vi "Untitled 21 (SubVI).vi"(6 "passband bandwidth (Hz)":dbl, 7 "pulse shaping filter (none) in":T1(ring), 9 "carrier frequency (Hz) in":dbl, 10 "Numeric":i32, 11 "passband waveform":waveform(dbl)) -> (3 "output bit stream":i8[](array[numeric]))   [LabVIEW 2017]
uses:
  <vilib>/addons/Modulation/Analog/support/mod_Set Error Source.vi
  <vilib>/addons/Modulation/Digital/General/MT Generate ASK system parameters (M).vi
  <vilib>/addons/Modulation/Digital/Support/Common/Validators/mod_Generate Filter Coefficients Validate.vi
  <vilib>/addons/Modulation/Digital/General/subVIs/mod_Generate Filter Coefficients.vi
  <vilib>/addons/Modulation/Analog/MT Downconvert Passband (Real).vi
  <vilib>/addons/Modulation/niDMT.lvlib
  <vilib>/addons/Modulation/niAMT.lvlib
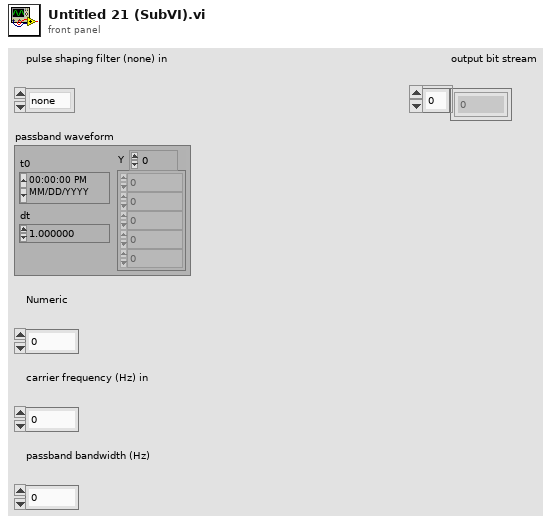
[diagram p1: front panel]
types:
  T1 = enum16{"none", "Raised Cosine", "Root Raised Cos", "Gaussian"}
  T2 = enum16{"FSK", "PSK", "QAM", "MSK", "PAM", "ASK", "CPM"}
  T3 = typedef "niAMT.lvlib/Complex Data Waveform.ctl" = cluster{"t0":dbl, "dt":dbl, "Y":cdb[]}
  T4 = cluster{"samples per symbol (16)":i32, "symbol map":cdb[]}
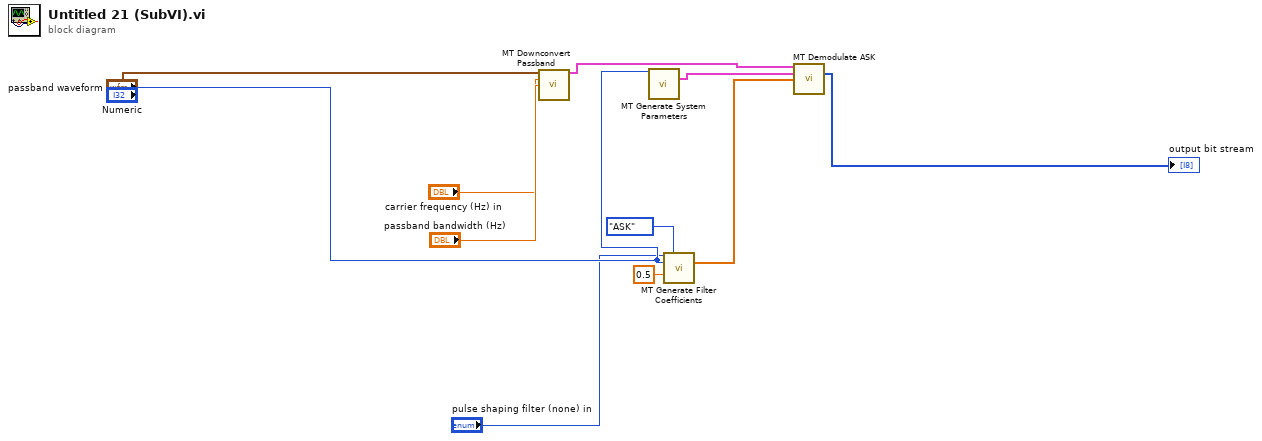
[diagram p0: block diagram]
diagram:
  n1 = call-poly <vilib>:"MT Downconvert Passband.vi"("Waveform"="passband waveform", "carrier frequency (Hz)"="carrier frequency (Hz) in", "passband bandwidth (Hz)"="passband bandwidth (Hz)") -> ("downconverted waveform (complex baseband)"=w11:T3)  [unwired: 9 in, 3 out]
  n2 = call-poly <vilib>:"MT Generate System Parameters.vi"("samples per symbol (16)"="Numeric") -> ("ASK system parameters"=w8:T4)  [unwired: 12 in, 2 out]
  n3 = call <vilib>:"MT Generate Filter Coefficients.vi"("pulse shaping filter (none)"="pulse shaping filter (none) in", "modulation type"=T2."ASK", "pulse shaping samples per symbol (16)"="Numeric", "filter parameter"=0.5) -> ("matched filter coefficients"=w6:dbl[])  [unwired: 9 in, 2 out]
  n4 = call <vilib>:"MT Demodulate ASK.vi"("input complex waveform"=w11, "ASK system parameters"=w8, "matched filter coefficients"=w6) -> ("output bit stream"=→"output bit stream":i8[])  [unwired: 8 in, 4 out]
